vi "Load JSON Match Numbers.vi"(10 "All Files in Dir":path[](array[path]), 11 "ListBox in":refnum<vi>) -> ()   [LabVIEW 2015]
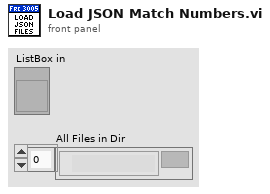
[diagram p1: front panel]
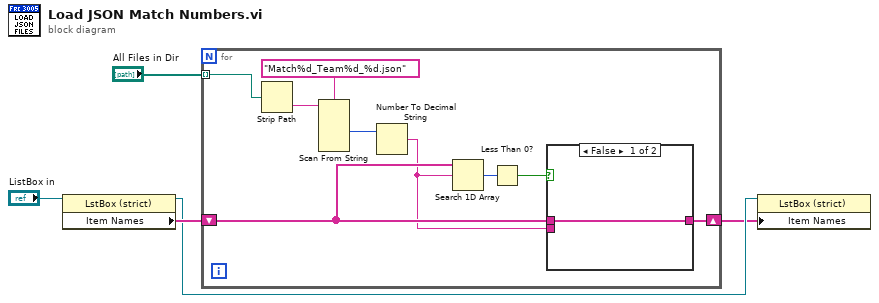
[diagram p0: block diagram]
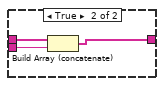
[diagram p2: hidden frame]
diagram:
  n1 = property class="LstBox (strict)"(reference="ListBox in") -> (reference out=w2:refnum<vi>, "Item Names"=w3:string[])  [unwired: 1 in, 1 out]
  n2 = for {
    tunnel: "All Files in Dir" -> [w14] mode=indexing
    shift-right: [w6] -> w1
    shift-left: w3 -> [w8]
    n3 = Strip Path(path=w14) -> (name=w13:string)  [unwired: 1 out]
    n4 = Scan From String(format string="Match%d_Team%d_%d.json", input string=w13) -> (output 1=w11:i32)  [unwired: 7 in, 3 out]
    n5 = Number To Decimal String(number=w11) -> (decimal integer string=w7:string)  [unwired: 1 in]
    n6 = Search 1D Array(1D array=w8, element=w7) -> (index of element=w10:i32)  [unwired: 1 in]
    n7 = Less Than 0?(x=w10) -> (x < 0?=w9:bool)
    n8 = case shown="False" w9 {
      tunnel: w8 -> [w15 w18]
      tunnel: w7 -> [_ w17]
      tunnel: [w15 w16] -> w6
      frame False {
      }
      frame True {
        n9 = Build Array (concatenate)(w18, w17) -> (w16:string[])
      }
    }
  }
  n10 = property class="LstBox (strict)"(reference=w2, "Item Names"=w1) -> ()  [unwired: 1 in, 2 out]
